vi "sliderstp.vi"(0 "y":dbl, 1 "Slide Ref":refnum<vi>) -> ()   [LabVIEW 2010]
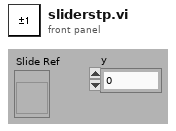
[diagram p1: front panel]
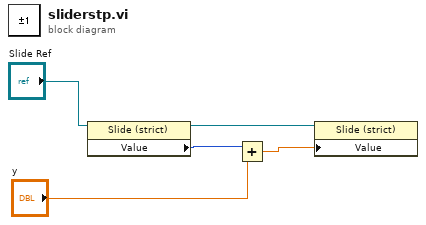
[diagram p0: block diagram]
diagram:
  n1 = property class="Slide (strict)"(reference="Slide Ref") -> (reference out=w4:refnum<vi>, "Value"=w3:u8)  [unwired: 1 in, 1 out]
  n2 = Add(x=w3, y="y") -> (x+y=w1:dbl)
  n3 = property class="Slide (strict)"(reference=w4, "Value"=w1) -> ()  [unwired: 1 in, 2 out]
